vi "NewProtocolEntry.vi"() -> (3 "ProtocolEntryT 2":T1 {"Zeitstempel" format=" %<%X %x>T"})   [LabVIEW 2014]
doc: "Erstellt neuen Protokoll Eintrag und gibt diesen zurück"
uses:
  controls/ProtocolEntry.ctl
panel:
  in  "Commit":bool
  in  "ProtocolEntryT":T1 {"Zeitstempel" format=" %<%X %x>T"}
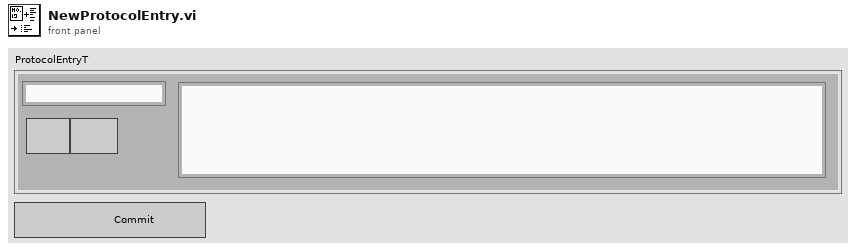
[diagram p1: front panel]
types:
  T1 = typedef "ProtocolEntry.ctl" = cluster{"Zeitstempel":timestamp, "String":string, "Abbrechen-Schaltfläche":bool, "Optionen-Schaltfläche":bool}
  T2 = cluster{"ProtocolEntryT":refnum<vi>, "Zeitstempel":refnum<vi>, "String":refnum<vi>}
  T3 = cluster{cluster{"ProtocolEntryT":refnum<vi>, "Zeitstempel":refnum<vi>, "String":refnum<vi>}, cluster{"Commit":refnum<vi>}}
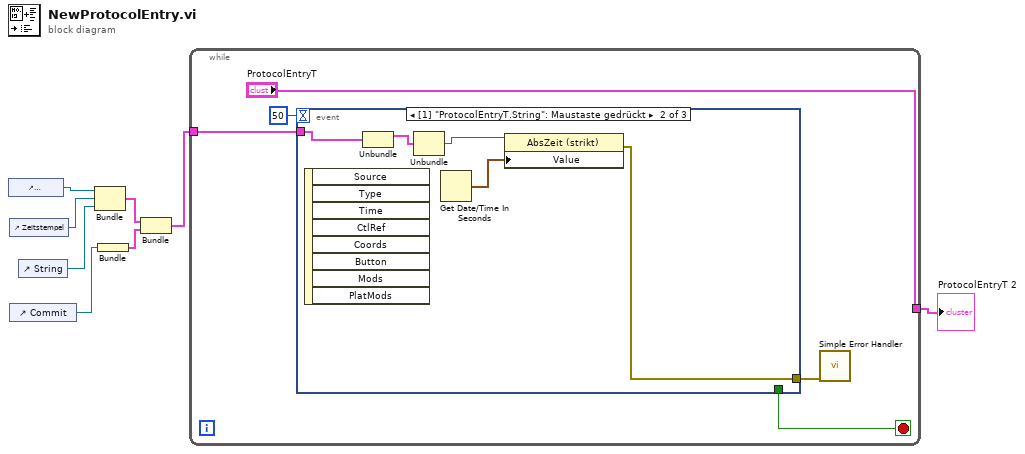
[diagram p0: block diagram]
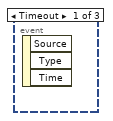
[diagram p2: hidden frame]
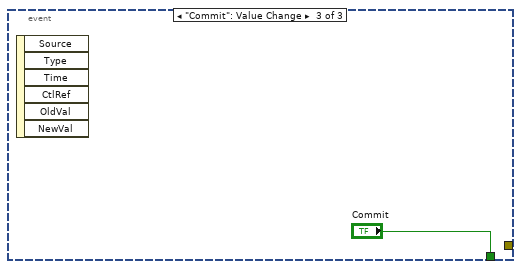
[diagram p3: hidden frame]
diagram:
  n1 = control-ref of="ProtocolEntryT"() -> (w8:refnum<vi>)
  n2 = control-ref of="Zeitstempel"() -> (w7:refnum<vi>)
  n3 = control-ref of="Commit"() -> (w5:refnum<vi>)
  n4 = control-ref of="String"() -> (w6:refnum<vi>)
  n5 = Bundle("ProtocolEntryT"=w8, "Zeitstempel"=w7, "String"=w6) -> (w4:T2)  [unwired: 1 in]
  n6 = Bundle("Commit"=w5) -> (w3:cluster{"Commit":refnum<vi>})  [unwired: 1 in]
  n7 = Bundle(w4, w3) -> (w2:T3)  [unwired: 1 in]
  n8 = while {
    tunnel: w2 -> [w13]
    tunnel: ["ProtocolEntryT"] -> w1
    stop <- w9 stop-if-true
    n9 = event shown="[1] \"ProtocolEntryT.String\": Maustaste gedrückt" {
      selector: _ -> [_ _ _]
      dyn-events: _ -> [_ _ _]
      timeout: 50 -> [_ _ _]
      tunnel: w13 -> [_ w18 _]
      tunnel: [_ w15 _] -> w12
      tunnel: [_ _ "Commit"] -> w9
      event Timeout {
        n10 = event-data() -> ()  [unwired: 1 in, 3 out]
      }
      event Mouse Down {
        n11 = event-data() -> ()  [unwired: 1 in, 8 out]
        n12 = Unbundle(w18) -> (w17:T2)  [unwired: 1 out]
        n13 = Unbundle(w17) -> ("Zeitstempel"=w16:refnum<vi>)  [unwired: 2 out]
        n14 = Get Date/Time In Seconds() -> (seconds since 1Jan1904=w14:timestamp)
        n15 = property class="AbsZeit (strikt)"(reference=w16, "Value"=w14) -> (error out=w15:errorcluster)  [unwired: 1 in, 1 out]
      }
      event "Commit": Value Change {
        n16 = event-data() -> ()  [unwired: 1 in, 6 out]
      }
    }
    n17 = call <vilib>:"Simple Error Handler.vi"("error in (no error)"=w12) -> ()  [unwired: 4 in, 5 out]
  }
  "ProtocolEntryT 2" <- w1
